vi "Check Complete.vi"(8 "error in (no error)":errorcluster, 11 "Burrow in":refnum<class "Burrow.lvclass">) -> (0 "error out":errorcluster, 2 "Complete?":bool, 3 "Burrow out":refnum<class "Burrow.lvclass">)   [LabVIEW 2019, in "23.lvlib" / "Burrow.lvclass"]
uses:
  Burrow.lvclass
  Amphipod/Amphipod.lvclass
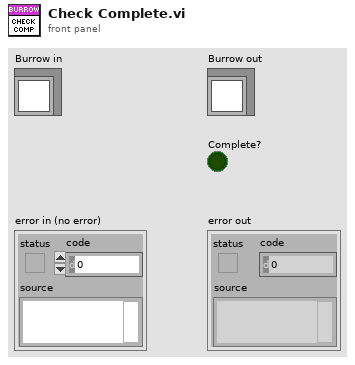
[diagram p1: front panel]
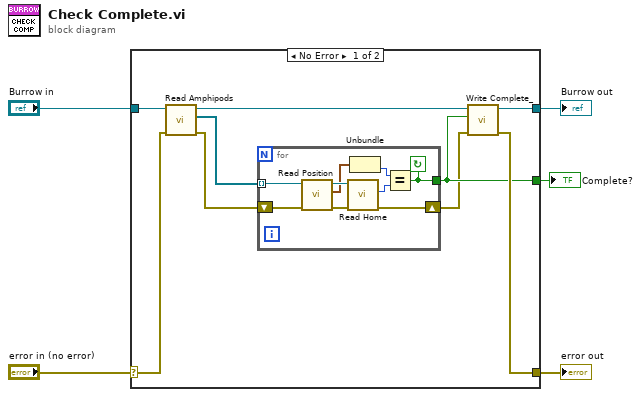
[diagram p0: block diagram]
diagram:
  n1 = case shown="No Error" "error in (no error)" {
    selector: "error in (no error)" -> [w13 w25]
    tunnel: [w10 w25] -> w4
    tunnel: [w11 w24] -> w2
    tunnel: "Burrow in" -> [w14 w24]
    tunnel: [w8 _] -> w1
    frame No Error {
      n2 = call-dynamic "Read Amphipods.vi"("error in (no error)"=w13, "Burrow in"=w14) -> ("error out"=w7:errorcluster, "Amphipods"=w9:refnum<class "Amphipod.lvclass">[], "Burrow out"=w12:refnum<class "Burrow.lvclass">)  [unwired: 7 in]
      n3 = for {
        tunnel: w9 -> [w23] mode=indexing
        tunnel: [w18] -> w8
        shift-right: [w15] -> w6
        shift-left: w7 -> [w16]
        stop <- w18 continue-if-true
        n4 = call-dynamic "Read Position.vi"("error in (no error)"=w16, "Amphipod in"=w23) -> ("error out"=w17:errorcluster, "Position"=w21:cluster{"Row":i8, "Column":i8}, "Amphipod out"=w22:refnum<class "Amphipod.lvclass">)  [unwired: 7 in]
        n5 = call-dynamic "Read Home.vi"("error in (no error)"=w17, "Amphipod in"=w22) -> ("error out"=w15:errorcluster, "Home"=w19:i8)  [unwired: 7 in, 1 out]
        n6 = Unbundle(w21) -> ("Column"=w20:i8)  [unwired: 1 out]
        n7 = Equal?(x=w20, y=w19) -> (x = y?=w18:bool)
      }
      n8 = call-dynamic "Write Complete_.vi"("error in (no error)"=w6, "Complete?"=w8, "Burrow in"=w12) -> ("error out"=w10:errorcluster, "Burrow out"=w11:refnum<class "Burrow.lvclass">)  [unwired: 7 in]
    }
    frame Error {
    }
  }
  "error out" <- w4
  "Burrow out" <- w2
  "Complete?" <- w1
